vi "Teleop.vi"(10 "Match Info":T1={"Autonomous Elapsed Seconds"=0.0, "TeleOp Elapsed Seconds"=108.644, "Disabled Elapsed Seconds"=9.52, "Visited Autonomous"=FALSE, "Visited TeleOp"=TRUE, "Visited Disabled"=TRUE, "Autonomous Settings"={"Autonomous Style"=enum."Independent", "VI Refnum"=refnum}}, 11 "Call Context":T2=enum."Stop") -> ()   [LabVIEW 2014]
doc: "This VI is called for each TeleOp packet received from the DS where the robot is not disabled. It is often used to read from the joysticks and update I/O or to update setpoints for timed control loops. It should complete and return within 20 milliseconds or it may miss DS packets."
uses:
  <vilib>/Rock Robotics/WPI/DriverStation/WPI_DriverStationDerivedRobotMode.ctl
  <vilib>/Rock Robotics/WPI/DriverStation/WPI_DriverStationMatch Info.ctl
  <vilib>/Rock Robotics/WPI/Joystick/WPI_JoystickGetSetRefNum.vi
  <vilib>/Rock Robotics/Network Tables/SD Read Boolean.vi
  <vilib>/Rock Robotics/Network Tables/SD Read Number.vi
panel:
  in  "Normal_Speed":dbl=1000.0
  in  "Top_Speed":dbl=2500.0
  out "Numeric":dbl format="%#_13g"
  in  "Rotation Gain":dbl=0.5
  out "Lift_2_Target":dbl=1781.283911323472
  in  "Integrate_Lift2_Output":bool=TRUE
  out "Lift2_Rate_Cmd":dbl=-0.0
  in  "Min_Lift2_Rate":dbl=-1000.0
  in  "Max_Lift2_Rate":dbl=1000.0
  in  "Integrate_Lift1_Output":bool=TRUE
  in  "Z_Deadband_Center":dbl format="%#_13g"
  in  "Z_Deadband_Size(%)":dbl=15.0 format="%#_13g"
  in  "Y_Deadband_Center":dbl format="%#_13g"
  in  "Y_Deadband_Size(%)":dbl=15.0 format="%#_13g"
  in  "X_Deadband_Center":dbl format="%#_13g"
  in  "X_Deadband_Size(%)":dbl=15.0 format="%#_13g"
  in  "Deadband_Center 2":dbl=-0.00784 format="%#_13g"
  in  "Deadband_Center":dbl=-0.00784 format="%#_13g"
  in  "Deadband_Size(%) 2":dbl=9.0 format="%#_13g"
  in  "Deadband_Size(%)":dbl=9.0 format="%#_13g"
  in  "Lift_2_Stick_Gain":dbl=40.0
  in  "Max_Lift_2_Target":dbl=3300.0
  in  "Min_Lift_2_Target":dbl=-100.0
  in  "Min_Lift_1_Target":dbl=-1.0
  in  "Max_Lift_1_Target":dbl=1.0
  in  "Lift_1_Stick_Gain":dbl=100.0
  out "Sample Slider 0":dbl(slide) scale=0.0..5.0
  out "Sample Boolean 1":bool
  out "Sample Boolean 0":bool
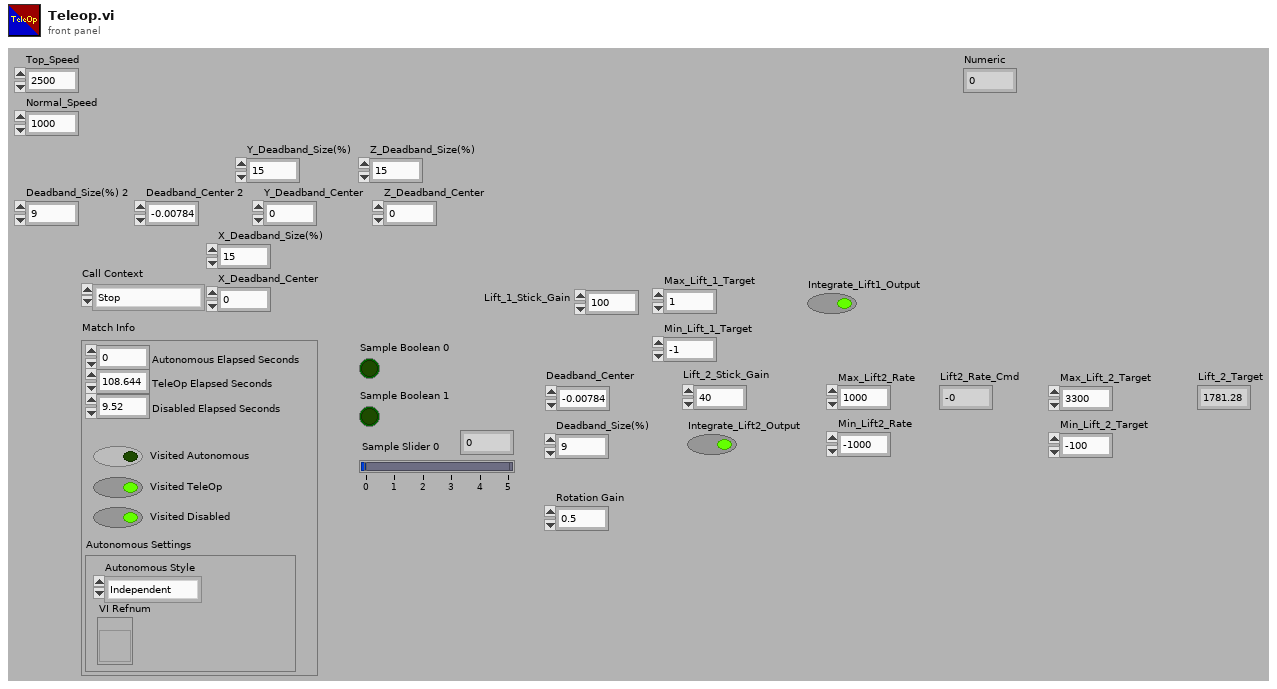
[diagram p1: front panel]
types:
  T1 = typedef "WPI_DriverStationMatch Info.ctl" = cluster{"Autonomous Elapsed Seconds":dbl, "TeleOp Elapsed Seconds":dbl, "Disabled Elapsed Seconds":dbl, "Visited Autonomous":bool, "Visited TeleOp":bool, "Visited Disabled":bool, "Autonomous Settings":cluster{"Autonomous Style":enum16{"Iterative", "Independent"}, "VI Refnum":refnum<vi>}}
  T2 = typedef "WPI_DriverStationDerivedRobotMode.ctl" = enum16{"Init", "Execute", "Stop"}
  T3 = typedef "WPI_JoystickDevRef.ctl" = cluster{"Device":T4}
  T4 = typedef "WPI_JoystickDeviceEnum.ctl" = enum16{"USB 0", "USB 1", "USB 2", "USB 3", "USB 4", "USB 5"}
  T5 = cluster{"Button 1":bool, "Button 2":bool, "Button 3":bool, "Button 4":bool, "Button 5":bool, "Button 6":bool, "Button 7":bool, "Button 8":bool, "Button 9":bool, "Button 10":bool, "Button 11":bool, "Button 12":bool}
  T6 = cluster{"axis 1 (x)":dbl, "axis 2 (y)":dbl, "axis 3 (throttle)":dbl, "axis 4":dbl, "axis 5":dbl, "axis 6":dbl}
  T7 = typedef "WPI_GyroDevRef.ctl" = cluster{"DevStatus":errorcluster, "Analog Module":T8, "Analog Channel":T9, "Offset":dbl, "Gain (VoltsPerDegree/Second)":dbl}
  T8 = typedef "FPGA_TypedefAnalogModule.ctl" = enum16{"Controller 1"}
  T9 = typedef "FPGA_AIChannel.ctl" = enum8{"AI 0", "AI 1", "AI 2", "AI 3", "AI MXP 0", "AI MXP 1", "AI MXP 2", "AI MXP 3", "Invalid"}
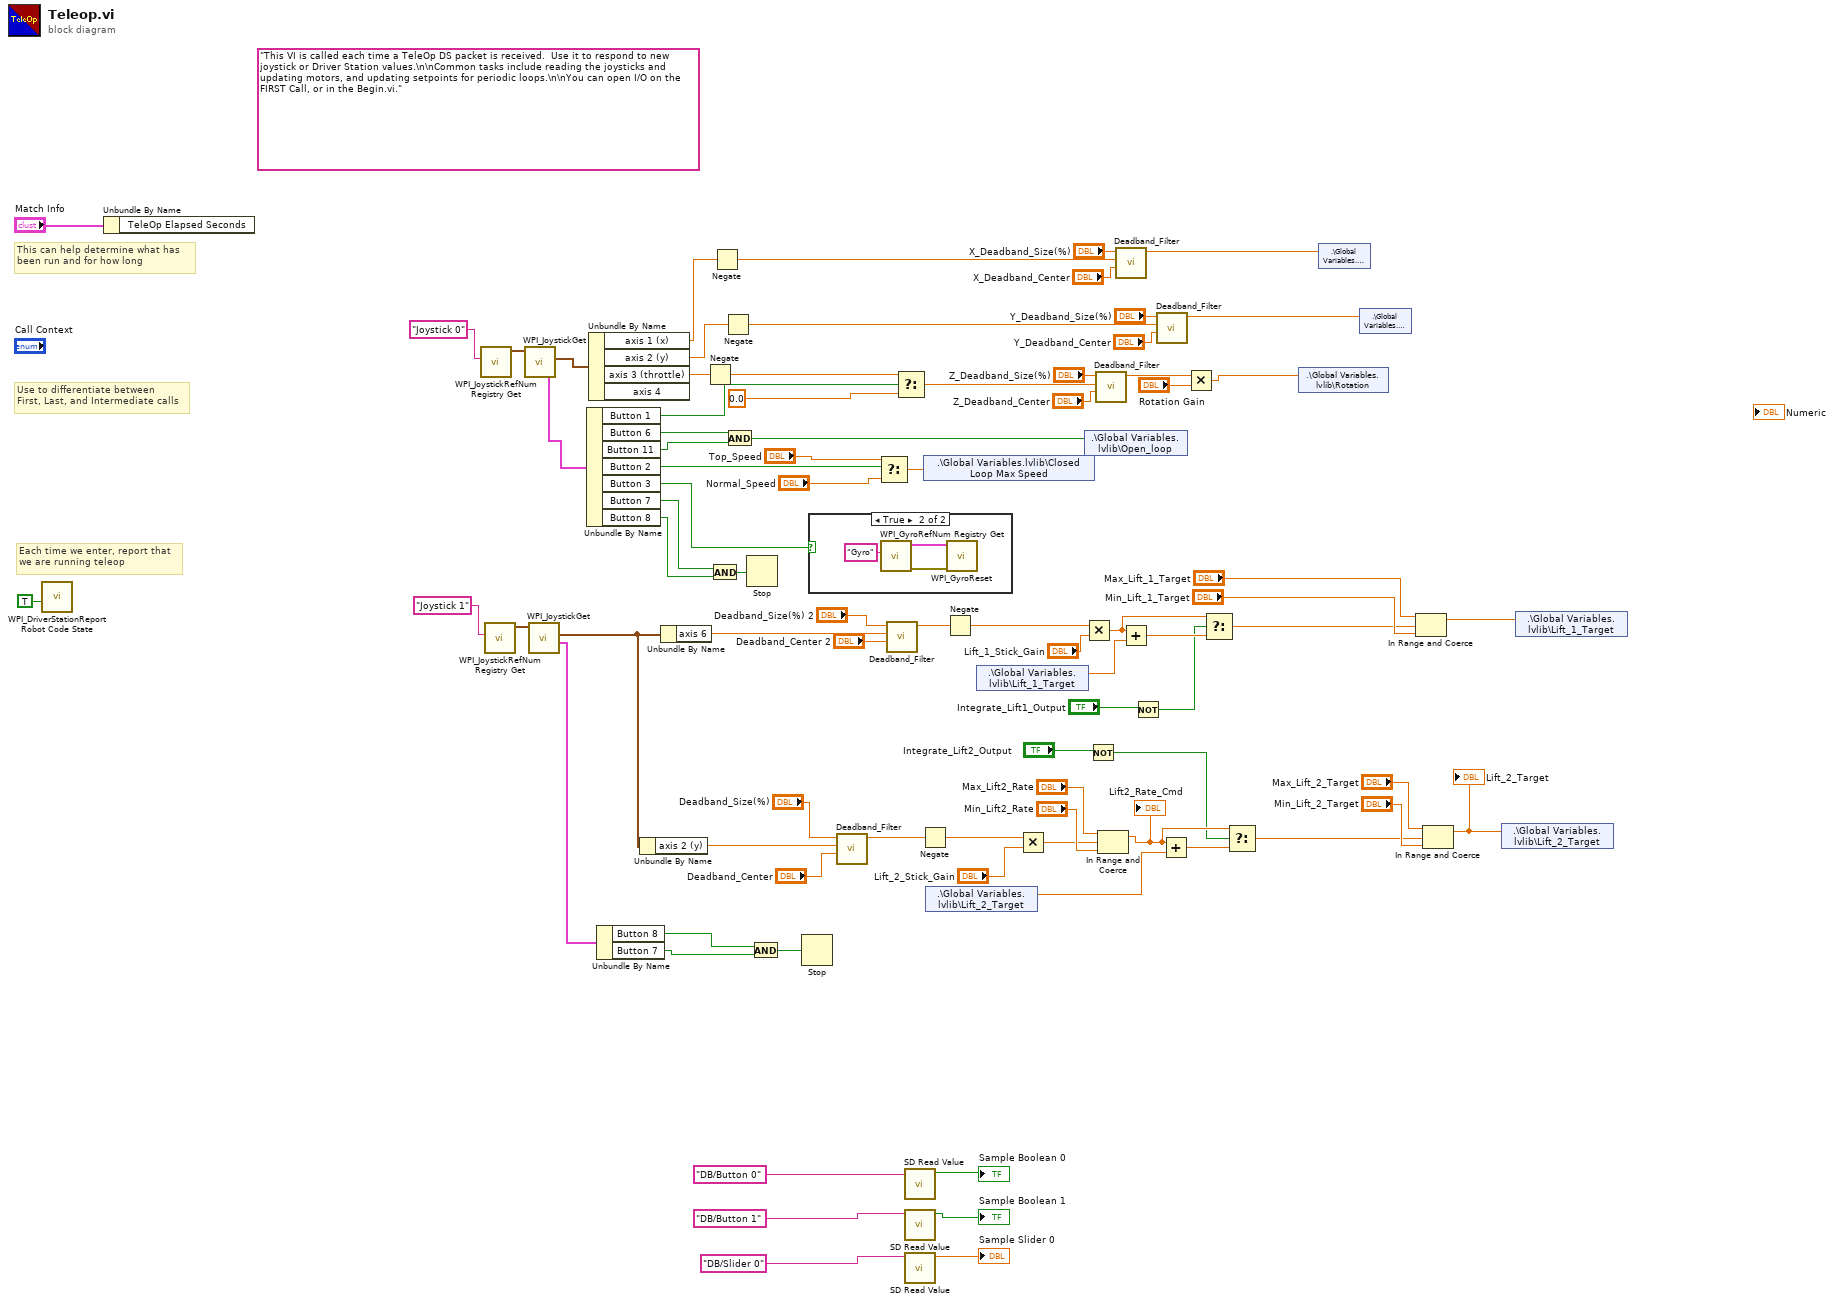
[diagram p0: block diagram]
diagram:
  (unwired) "This VI is called each time a TeleOp DS packet is received.  Use it to respond to new joystick or Driver Station values.\n\nCommon tasks include reading the joysticks and updating motors, and updating setpoints for periodic loops.\n\nYou can open I/O on the FIRST Call, or in the Begin.vi."
  # "Each time we enter, report that\nwe are running teleop"
  # "Use to differentiate between\nFirst, Last, and Intermediate calls"
  # "This can help determine what has\nbeen run and for how long"
  n1 = call <vilib>:"WPI_DriverStationReport Robot Code State.vi"("TeleOp"=TRUE ("Autonomous")) -> ()  [unwired: 10 in, 1 out]
  n2 = Unbundle By Name("Match Info") -> ()  [unwired: 1 out]
  n3 = call <vilib>:"WPI_JoystickRefNum Registry Get.vi"("refnum name"="Joystick 0") -> ("JoystickDevRef"=w74:T3)  [unwired: 1 in, 9 out]
  n4 = call <vilib>:"WPI_JoystickRefNum Registry Get.vi"("refnum name"="Joystick 1") -> ("JoystickDevRef"=w71:T3)  [unwired: 1 in, 9 out]
  n5 = call <vilib>:"WPI_JoystickGet.vi"("JoystickDevRef"=w74) -> ("Buttons"=w70:T5, "Axes"=w73:T6)  [unwired: 1 in, 4 out]
  n6 = call <vilib>:"WPI_JoystickGet.vi"("JoystickDevRef"=w71) -> ("Buttons"=w4:T5, "Axes"=w66:T6)  [unwired: 1 in, 4 out]
  n7 = Unbundle By Name(w70) -> ("Button 1"=w67:bool, "Button 6"=w21:bool, "Button 11"=w20:bool, "Button 2"=w11:bool, "Button 3"=w12:bool, "Button 7"=w7:bool, "Button 8"=w6:bool)
  n8 = Unbundle By Name(w73) -> ("axis 1 (x)"=w48:dbl, "axis 2 (y)"=w46:dbl, "axis 3 (throttle)"=w69:dbl)  [unwired: 1 out]
  n9 = Unbundle By Name(w4) -> ("Button 8"=w2:bool, "Button 7"=w3:bool)
  n10 = Unbundle By Name(w66) -> ("axis 2 (y)"=w53:dbl)
  n11 = Unbundle By Name(w66) -> ("axis 6"=w55:dbl)
  n12 = Negate(x=w69) -> (-x=w16:dbl)
  n13 = And(x=w7, y=w6) -> (x .and. y?=w5:bool)
  n14 = Negate(x=w48) -> (-x=w18:dbl)
  n15 = Negate(x=w46) -> (-x=w17:dbl)
  n16 = And(x=w21, y=w20) -> (x .and. y?=w19:bool)
  n17 = Stop(stop? (T)=w5) -> ()
  n18 = And(x=w2, y=w3) -> (x .and. y?=w1:bool)
  n19 = Stop(stop? (T)=w1) -> ()
  n20 = case shown="True" w12 {
    frame False {
    }
    frame True {
      n21 = call <vilib>:"WPI_GyroRefNum Registry Get.vi"("refnum name"="Gyro") -> ("error out"=w85:errorcluster, "GyroDevRef"=w84:T7)  [unwired: 9 in]
      n22 = call <vilib>:"WPI_GyroReset.vi"("error in (no error)"=w85, "GyroDevRef"=w84) -> ()  [unwired: 8 in, 2 out]
    }
  }
  n23 = call "Deadband_Filter.vi"("Deadband_Center"="Deadband_Center", "Input"=w53, "Deadband_Size(%)"="Deadband_Size(%)") -> ("Deadbanded_Output"=w23:dbl)  [unwired: 8 in]
  n24 = Select(t="Top_Speed", s=w11, f="Normal_Speed") -> (s? t:f=w8:dbl)
  n25 = call "Deadband_Filter.vi"("Deadband_Center"="Deadband_Center 2", "Input"=w55, "Deadband_Size(%)"="Deadband_Size(%) 2") -> ("Deadbanded_Output"=w54:dbl)  [unwired: 8 in]
  n26 = Select(t=w16, s=w67, f=0.0) -> (s? t:f=w44:dbl)
  n27 = call-poly <vilib>:"SD Read Value.vi"("Name"="DB/Button 0" ("refnum name")) -> ("Boolean"=→"Sample Boolean 0":bool)  [unwired: 8 in, 2 out]
  n28 = call-poly <vilib>:"SD Read Value.vi"("Name"="DB/Button 1" ("refnum name")) -> ("Boolean"=→"Sample Boolean 1":bool)  [unwired: 8 in, 2 out]
  n29 = call-poly <vilib>:"SD Read Value.vi"("Name"="DB/Slider 0" ("refnum name")) -> ("Numeric"=→"Sample Slider 0":dbl)  [unwired: 8 in, 2 out]
  n30 = Negate(x=w23) -> (-x=w22:dbl)
  n31 = shared-variable ".\\Global Variables.lvlib\\Closed Loop Max Speed"(w8) -> ()  [unwired: 1 in, 1 out]
  n32 = shared-variable ".\\Global Variables.lvlib\\Lift_2_Target"() -> (w56:dbl)  [unwired: 1 in, 1 out]
  n33 = Negate(x=w54) -> (-x=w32:dbl)
  n34 = shared-variable ".\\Global Variables.lvlib\\Lift_1_Target"() -> (w57:dbl)  [unwired: 1 in, 1 out]
  n35 = Multiply(x=w22, y="Lift_2_Stick_Gain") -> (x*y=w29:dbl)
  n36 = Multiply(x=w32, y="Lift_1_Stick_Gain") -> (x*y=w35:dbl)
  n37 = shared-variable ".\\Global Variables.lvlib\\Open_loop"(w19) -> ()  [unwired: 1 in, 1 out]
  n38 = Not(x="Integrate_Lift2_Output") -> (.not. x?=w24:bool)
  n39 = call "Deadband_Filter.vi"("Deadband_Center"="Z_Deadband_Center", "Input"=w44, "Deadband_Size(%)"="Z_Deadband_Size(%)") -> ("Deadbanded_Output"=w15:dbl)  [unwired: 8 in]
  n40 = In Range and Coerce(upper limit="Max_Lift2_Rate", x=w29, lower limit="Min_Lift2_Rate") -> (coerced(x)=w28:dbl)  [unwired: 1 out]
  "Lift2_Rate_Cmd" <- w28
  n41 = call "Deadband_Filter.vi"("Deadband_Center"="X_Deadband_Center", "Input"=w18, "Deadband_Size(%)"="X_Deadband_Size(%)") -> ("Deadbanded_Output"=w47:dbl)  [unwired: 8 in]
  n42 = Add(x=w35, y=w57) -> (x+y=w37:dbl)
  n43 = Not(x="Integrate_Lift1_Output") -> (.not. x?=w26:bool)
  n44 = call "Deadband_Filter.vi"("Deadband_Center"="Y_Deadband_Center", "Input"=w17, "Deadband_Size(%)"="Y_Deadband_Size(%)") -> ("Deadbanded_Output"=w45:dbl)  [unwired: 8 in]
  n45 = Add(x=w28, y=w56) -> (x+y=w34:dbl)
  n46 = Multiply(x=w15, y="Rotation Gain") -> (x*y=w14:dbl)
  n47 = Select(t=w35, s=w26, f=w37) -> (s? t:f=w36:dbl)
  n48 = Select(t=w28, s=w24, f=w34) -> (s? t:f=w33:dbl)
  n49 = shared-variable ".\\Global Variables.lvlib\\Rotation"(w14) -> ()  [unwired: 1 in, 1 out]
  n50 = shared-variable ".\\Global Variables.lvlib\\X"(w47) -> ()  [unwired: 1 in, 1 out]
  n51 = shared-variable ".\\Global Variables.lvlib\\Y"(w45) -> ()  [unwired: 1 in, 1 out]
  n52 = In Range and Coerce(upper limit="Max_Lift_1_Target", x=w36, lower limit="Min_Lift_1_Target") -> (coerced(x)=w62:dbl)  [unwired: 1 out]
  n53 = In Range and Coerce(upper limit="Max_Lift_2_Target", x=w33, lower limit="Min_Lift_2_Target") -> (coerced(x)=w58:dbl)  [unwired: 1 out]
  "Lift_2_Target" <- w58
  n54 = shared-variable ".\\Global Variables.lvlib\\Lift_2_Target"(w58) -> ()  [unwired: 1 in, 1 out]
  n55 = shared-variable ".\\Global Variables.lvlib\\Lift_1_Target"(w62) -> ()  [unwired: 1 in, 1 out]
